vi "RelStatus.vi"(0 "VisaCluster":T1, 11 "error in (no error)":errorcluster) -> (4 "VisaCluster":T1, 6 "Display":string, 8 "Answer":string, 10 "Rel":bool, 15 "error out":errorcluster)   [LabVIEW 2014, in "FH 55.lvlib"]
doc: "Dieses VI zeigt ob die Relative-Funktion eingeschaltet oder ausgeschaltet ist.\n\nThis VI shows that the relative function is turned on or off."
uses:
  FH 55.lvlib
  TypeDef/VisaCluster.ctl
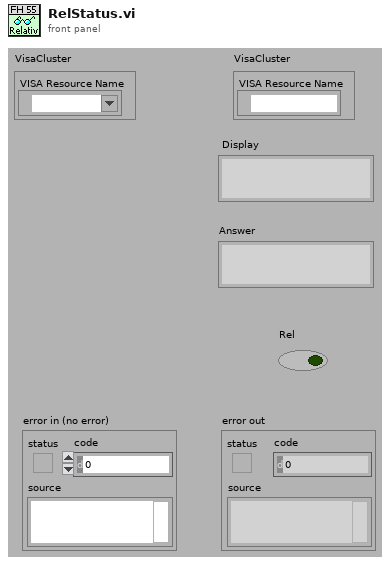
[diagram p1: front panel]
types:
  T1 = typedef "FH 55.lvlib/VisaCluster.ctl" = cluster{"VISA Resource Name":refnum<visa-resource-name>}
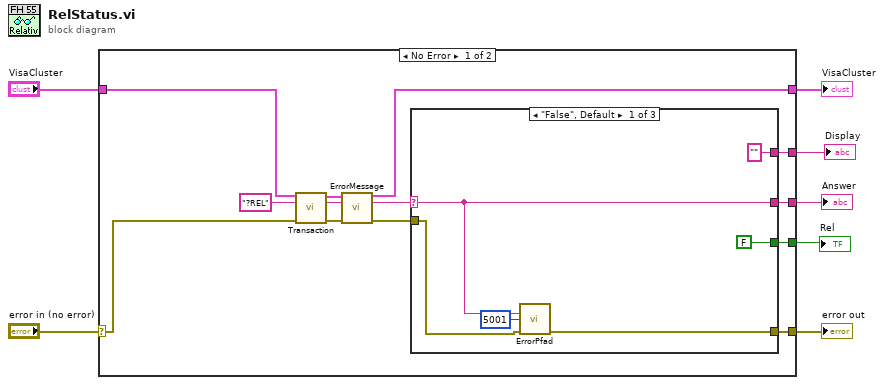
[diagram p0: block diagram]
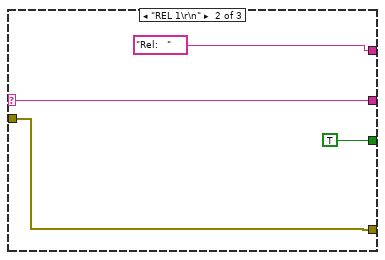
[diagram p2: hidden frame]
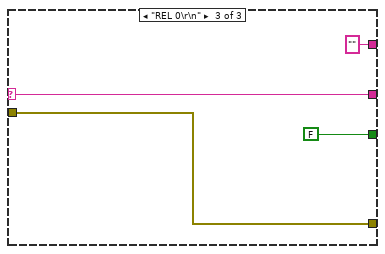
[diagram p3: hidden frame]
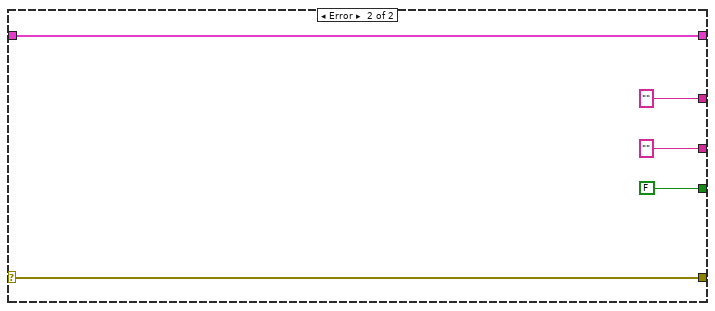
[diagram p4: hidden frame]
diagram:
  n1 = case shown="No Error" "error in (no error)" {
    selector: "error in (no error)" -> [w9 w38]
    tunnel: "VisaCluster" -> [w8 w39]
    tunnel: [w10 w39] -> w3
    tunnel: [w15 w38] -> w5
    tunnel: [w14 ""] -> w4
    tunnel: [w17 FALSE] -> w2
    tunnel: [w11 ""] -> w1
    frame No Error {
      n2 = call "Transaction.vi"("VisaCluster"=w8, "Command"="?REL", "error in (no error)"=w9) -> ("VisaCluster"=w19:T1, "Answer"=w12:string, "error out"=w20:errorcluster)  [unwired: 9 in, 1 out]
      n3 = call "ErrorMessage.vi"("VisaCluster"=w19, "Message In"=w12, "error in (no error)"=w20) -> ("VisaCluster"=w10:T1, "Message Out"=w13:string, "error out"=w16:errorcluster)  [unwired: 10 in]
      n4 = case shown="\"False\", Default" w13 {
        selector: w13 -> [w22 w29 w33]
        tunnel: [FALSE TRUE FALSE] -> w17
        tunnel: w16 -> [w25 w28 w32]
        tunnel: [w24 w28 w32] -> w15
        tunnel: [w22 w29 w33] -> w14
        tunnel: ["" "Rel:   " ""] -> w11
        frame "False", Default {
          n5 = call "ErrorPfad.vi"("Message In"=w22, "Numeric"=5001, "error in (no error)"=w25) -> ("error out"=w24:errorcluster)  [unwired: 11 in, 1 out]
        }
        frame "REL 1\r\n" {
        }
        frame "REL 0\r\n" {
        }
      }
    }
    frame Error {
    }
  }
  "error out" <- w5
  "Answer" <- w4
  "VisaCluster" <- w3
  "Rel" <- w2
  "Display" <- w1
